vi "Get Target Temperature.vi"(8 "error in":errorcluster, 11 "TEC 1090 in":refnum<class "Meerstetter TEC.lvclass">) -> (0 "error out":errorcluster, 2 "Number":sgl=92.92 format="%.10f", 3 "TEC 1090 out":refnum<class "Meerstetter TEC.lvclass">)   [LabVIEW 2014, in "Meerstetter Lib.lvlib" / "Meerstetter TEC.lvclass"]
uses:
  Meerstetter TEC.lvclass
  Controls/Read Parameters.ctl
  reusable/Session APIs/Serial/Serial Session.lvclass
  Meerstetter TEC.lvclass/Meerstetter TEC.ctl
  reusable/Session APIs/Serial/Public/Asynchronous Write.vi
  reusable/Session APIs/Serial/Public/Asynchronous Read.vi
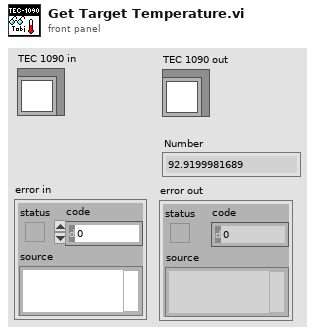
[diagram p1: front panel]
types:
  T1 = typedef "Meerstetter Lib.lvlib/Meerstetter TEC.lvclass/Read Parameters.ctl" = u16
  T2 = typedef "Session - Root.lvclass/Session Handle.ctl" = refnum<data-value>
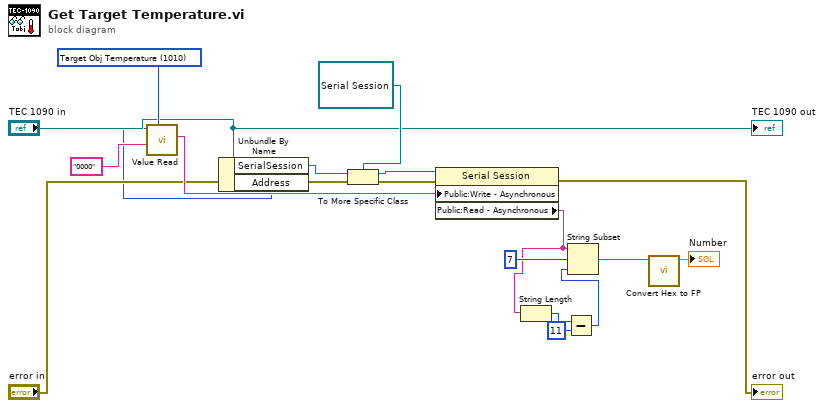
[diagram p0: block diagram]
diagram:
  w18 = T1 1010 items=["Device Type"=100, "Hardware Version"=101, "Serial Number"=102, "Firmware Version"=103, "Device Status"=104, "Error Number"=105, "Error Instance"=106, "Error Parameter"=107, "Save Data to Flash"=108, "Flash Status"=109, "Object Temperature"=1000, "Sink Temperature"=1001, "Target Obj Temperature"=1010, "Nominal Obj Temperature"=1011, "Thermal Power Mod Current"=1012, "Actual Output Current"=1020, "Actual Output Voltage"=1021, "Relative Cooling Power"=1100, "Nominal Fan Speed"=1101, "Actual Fan Speed"=1102, "Fan PWM Level"=1103, "PID Lower Limitation"=1030, "PID Upper Limitation"=1031, "PID Control Variable"=1032, "Obj Sensor Raw ADC Val"=1040, "Sink Sensor Raw ADC Val"=1041, "Object Sensor Resistance"=1042, "Sink Sensor Resistance"=1043, "Driver Input Voltage"=1060, "10V Internal Supply"=1061, "3.3V Internal Supply"=1062, "Base Plate Temperature"=1063, "Error Number"=1070, "Error Instance"=1071, "Error Parameter"=1072, "Temperature is Stable"=1200] ("Read Values")
  n1 = Unbundle By Name("TEC 1090 in") -> ("SerialSession"=w10:T2, "Address"=w1:u8)
  n2 = call "Value Read.vi"("Read Values"=w18, "Sequence"="0000", "Address"=w1) -> ("hex integer string"=w6:string)  [unwired: 8 in]
  n3 = To More Specific Class(target class=refnum<data-value> refnum, reference=w10, error in="error in") -> (specific class reference=w8:refnum<data-value>, error out=w4:errorcluster)
  n4 = property class="Serial Session"(reference=w8, error in=w4, "Public:Write - Asynchronous"=w6) -> (error out=→"error out":errorcluster, "Public:Read - Asynchronous"=w7:string)  [unwired: 1 out]
  n5 = String Length(string=w7) -> (length=w14:i32)
  n6 = Subtract(x=w14, y=11) -> (x-y=w12:i32)
  n7 = String Subset(string=w7, offset (0)=7, length (rest)=w12) -> (substring=w15:string)
  n8 = call "Convert Hex to FP.vi"("Hex String In"=w15) -> ("Number"=→"Number":sgl)  [unwired: 10 in]
  "TEC 1090 out" <- "TEC 1090 in"
